vi "virtualDS.vi"(4 "DS Digital Ins":T4, 6 "DS Analog Ins":T3 {"Analog 4" scale=0.0..65535.0; "Analog 3" scale=0.0..65535.0; "Analog 2" scale=0.0..65535.0; "Analog 1" scale=0.0..65535.0}, 7 "Control Byte":T2, 8 "JS 4":T5 {"Axes"."Axis 6" scale=-127.0..127.0; "Axes"."Axis 5" scale=-127.0..127.0; "Axes"."Axis 4" scale=-127.0..127.0; "Axes"."Axis 3" scale=-127.0..127.0; "Axes"."Axis 2" scale=-127.0..127.0; "Axes"."Axis 1" scale=-127.0..127.0}, 9 "JS 3":T5 {"Axes"."Axis 6" scale=-127.0..127.0; "Axes"."Axis 5" scale=-127.0..127.0; "Axes"."Axis 4" scale=-127.0..127.0; "Axes"."Axis 3" scale=-127.0..127.0; "Axes"."Axis 2" scale=-127.0..127.0; "Axes"."Axis 1" scale=-127.0..127.0}, 10 "JS 2":T5 {"Axes"."Axis 6" scale=-127.0..127.0; "Axes"."Axis 5" scale=-127.0..127.0; "Axes"."Axis 4" scale=-127.0..127.0; "Axes"."Axis 3" scale=-127.0..127.0; "Axes"."Axis 2" scale=-127.0..127.0; "Axes"."Axis 1" scale=-127.0..127.0}, 11 "JS 1":T5 {"Axes"."Axis 6" scale=-127.0..127.0; "Axes"."Axis 5" scale=-127.0..127.0; "Axes"."Axis 4" scale=-127.0..127.0; "Axes"."Axis 3" scale=-127.0..127.0; "Axes"."Axis 2" scale=-127.0..127.0; "Axes"."Axis 1" scale=-127.0..127.0}) -> ()   [LabVIEW 2011]
uses:
  joystick.ctl
panel:
  in  "IP Control":T1 {"Team Number" format="%04.0f"}
  out "Packet":string
  out "FRCCommonControlData":string
  out "Packet Number":u16
  in  "stop":bool
  out "length":i32
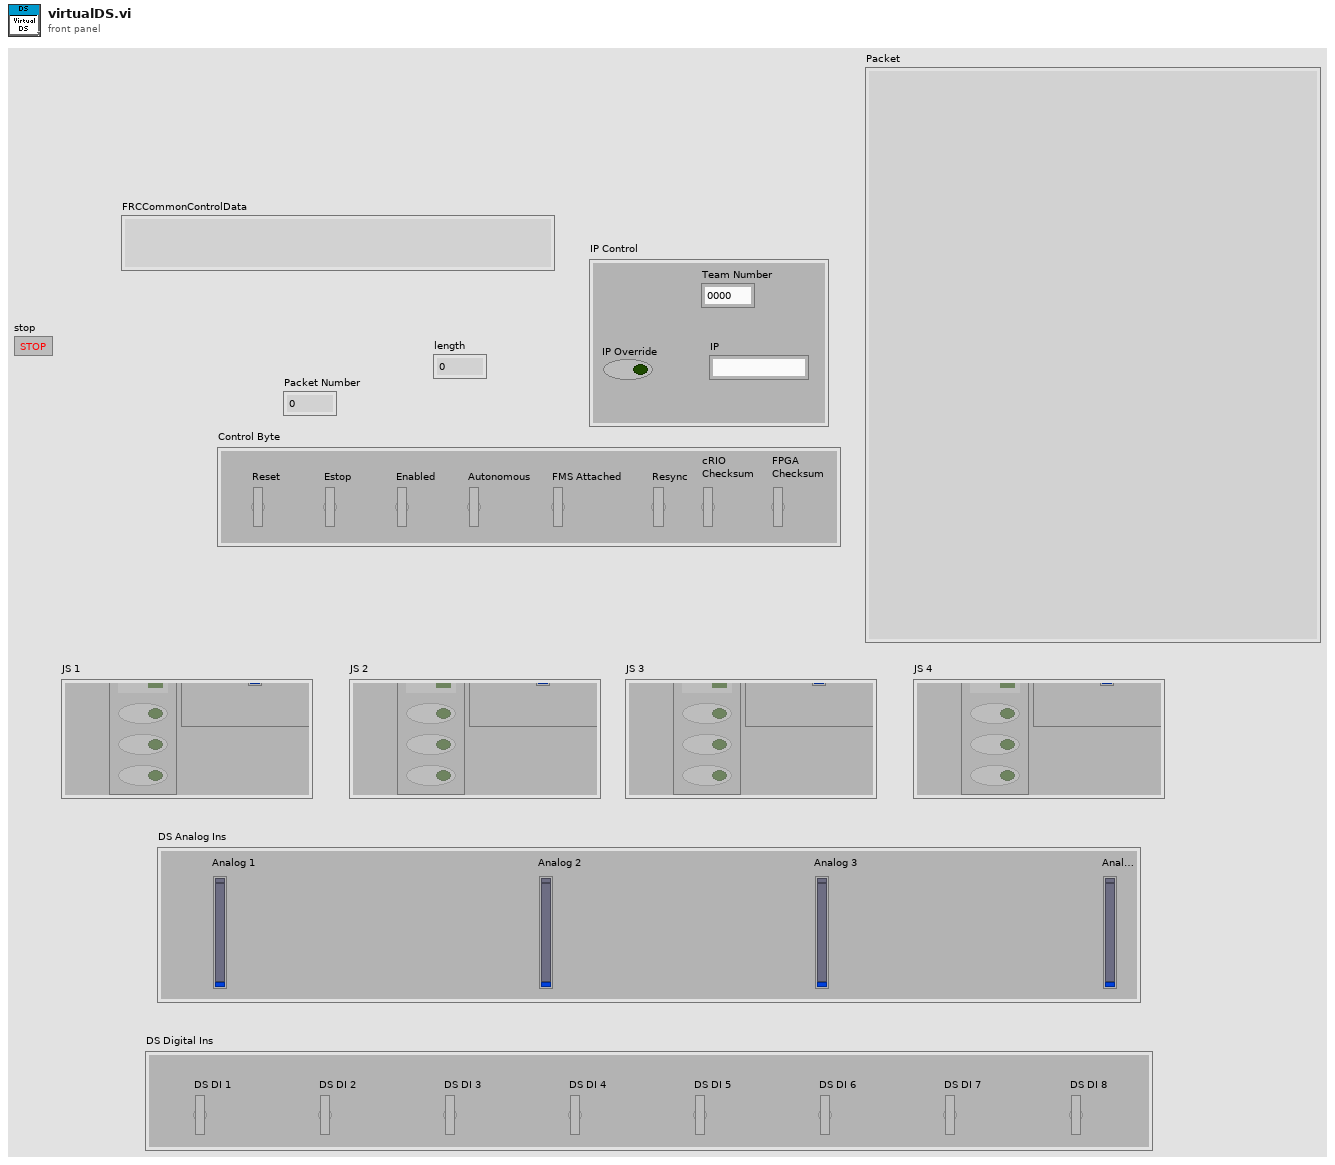
[diagram p1: front panel]
types:
  T1 = cluster{"Team Number":u16, "IP":string, "IP Override":bool}
  T2 = cluster{"Reset":bool, "Estop":bool, "Enabled":bool, "Autonomous":bool, "FMS Attached":bool, "Resync":bool, "cRIO \nChecksum":bool, "FPGA \nChecksum":bool}
  T3 = cluster{"Analog 1":u16, "Analog 2":u16, "Analog 3":u16, "Analog 4":u16}
  T4 = cluster{"DS DI 1":bool, "DS DI 2":bool, "DS DI 3":bool, "DS DI 4":bool, "DS DI 5":bool, "DS DI 6":bool, "DS DI 7":bool, "DS DI 8":bool}
  T5 = typedef "joystick.ctl" = cluster{"Axes":cluster{"Axis 1":u8, "Axis 2":u8, "Axis 3":u8, "Axis 4":u8, "Axis 5":u8, "Axis 6":u8}, "Buttons":bool[]}
  T6 = cluster{"Axis 1":u8, "Axis 2":u8, "Axis 3":u8, "Axis 4":u8, "Axis 5":u8, "Axis 6":u8}
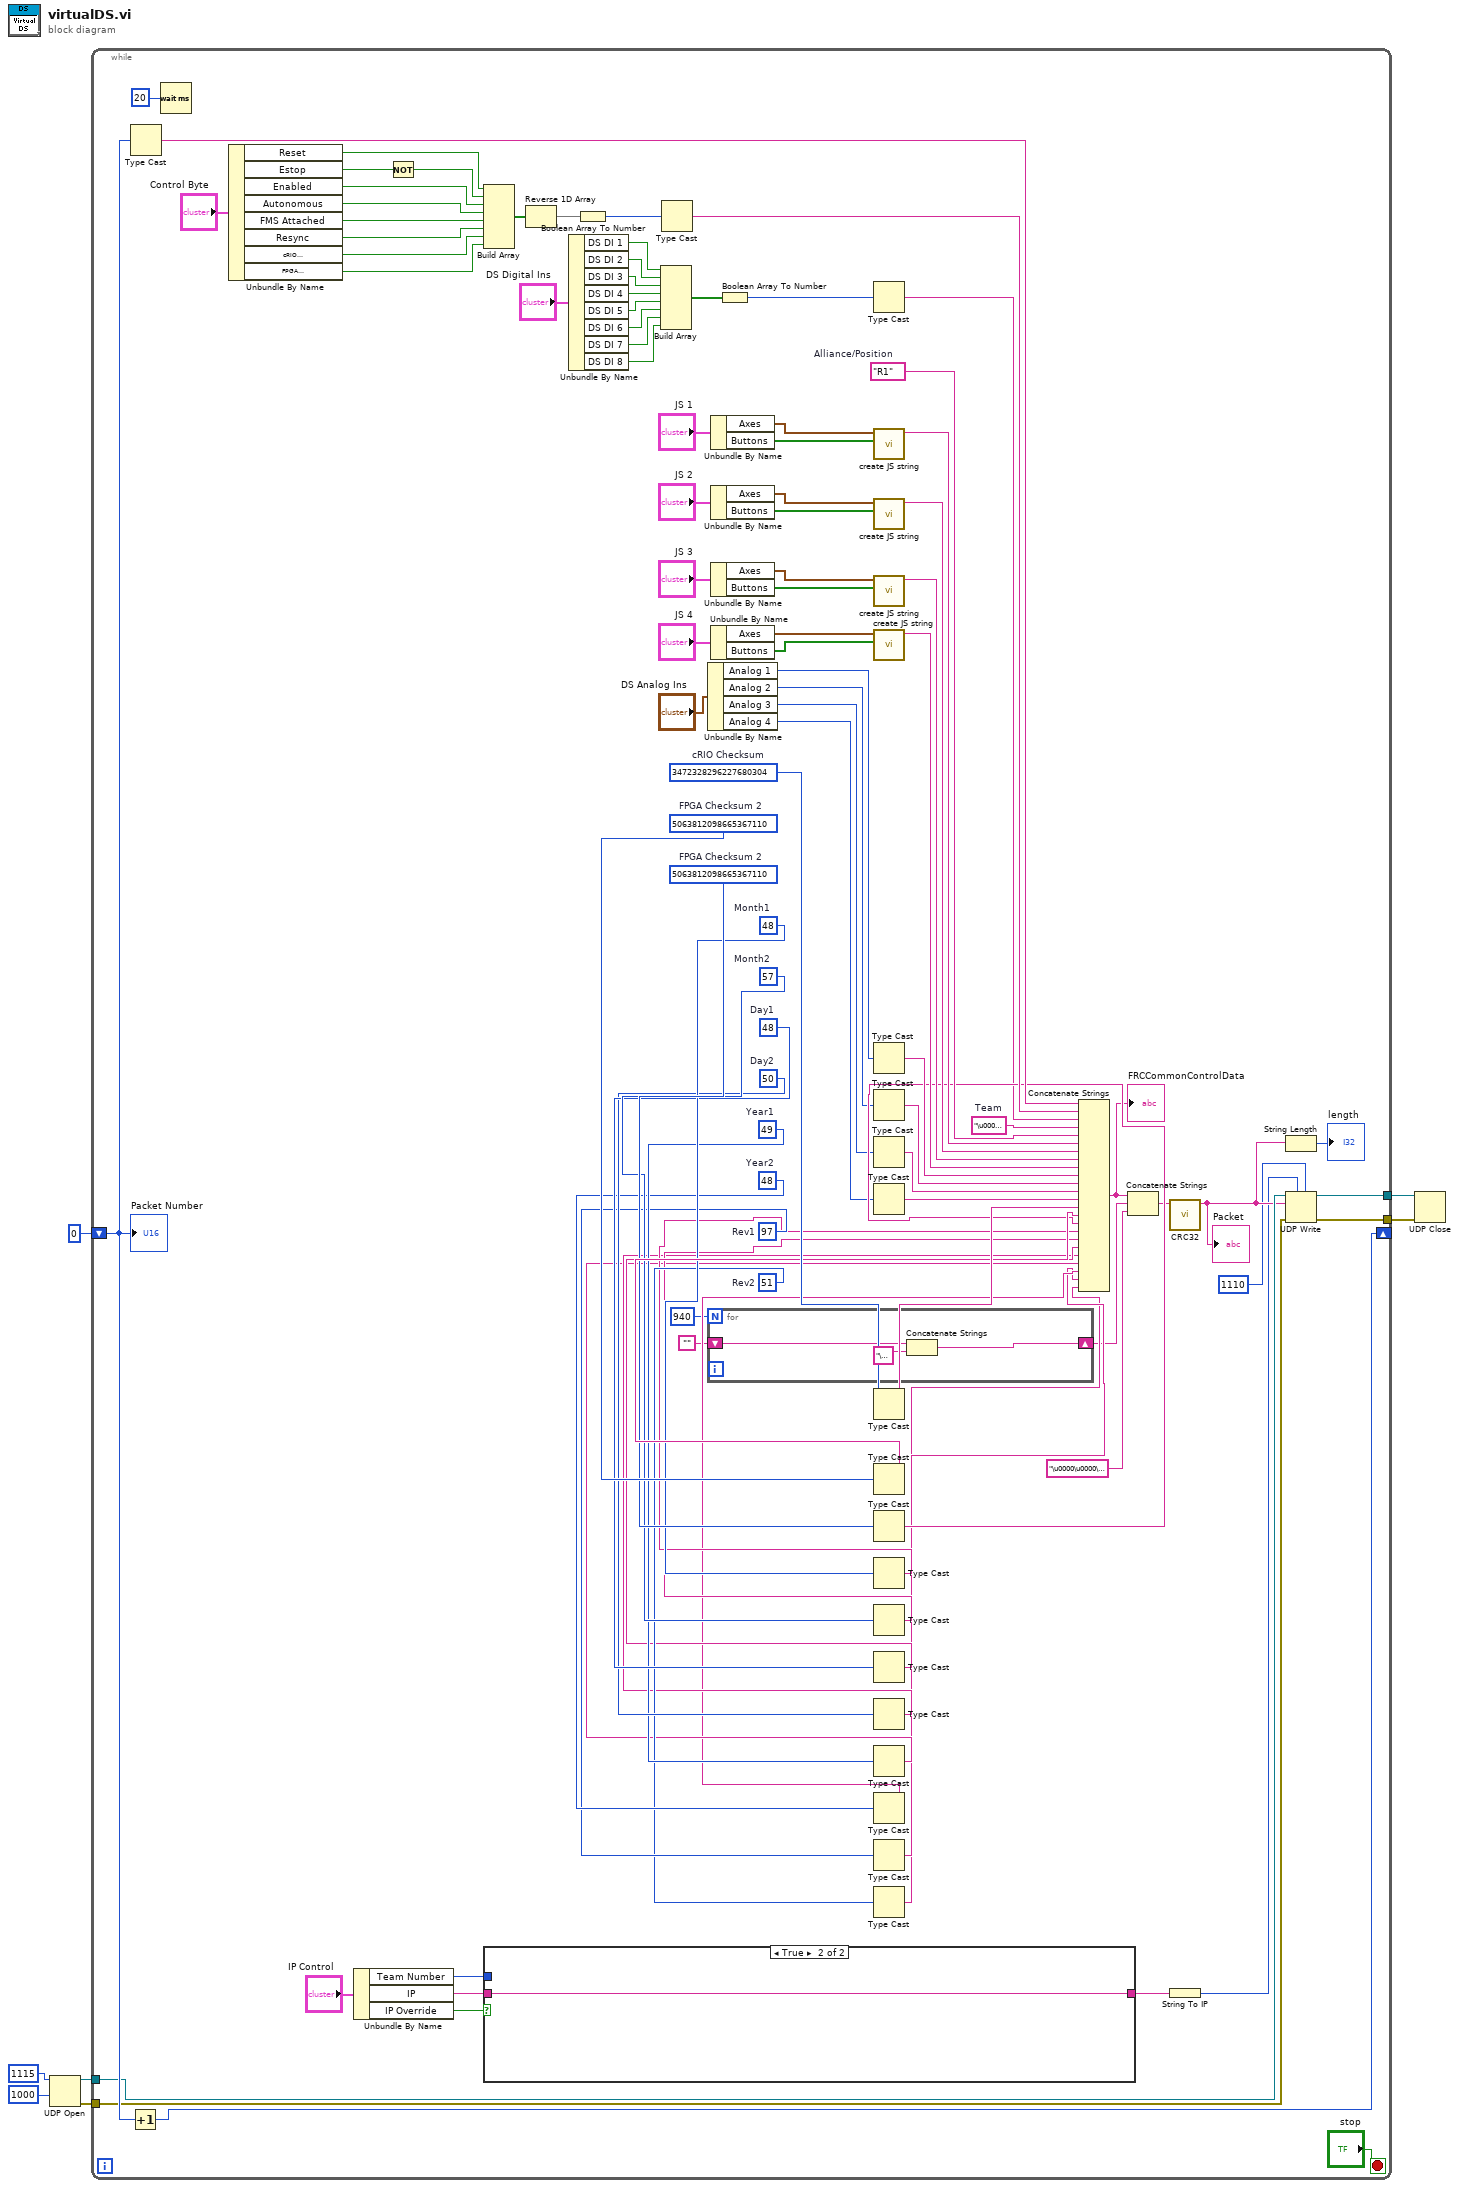
[diagram p0: block diagram]
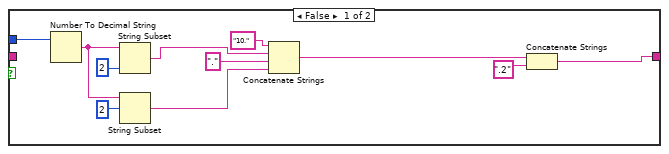
[diagram p2: hidden frame]
diagram:
  n1 = UDP Open(9:1000 ("timeout ms (25000)"), 11:u16 1115 ("port")) -> (port=w4:refnum<k16>, 0:w3:errorcluster)  [unwired: 3 in, 1 out]
  n2 = while {
    shift-right: [w106] -> _
    shift-left: u16 0 -> [w47]
    tunnel: w4 -> [w19]
    tunnel: w3 -> [w18]
    tunnel: [w16] -> w2
    tunnel: [w15] -> w1
    stop <- "stop" stop-if-true
    w66 = u8 51  # Rev2
    w67 = u8 97  # Rev1
    w68 = u8 48  # Year2
    w69 = u8 49  # Year1
    w70 = u8 50  # Day2
    w71 = u8 48  # Day1
    w72 = u8 57  # Month2
    w73 = u8 48  # Month1
    w75 = u64 5063812098665367110  # FPGA Checksum 2
    w77 = u64 5063812098665367110  # FPGA Checksum 2
    w79 = u64 3472328296227680304  # cRIO Checksum
    w100 = "R1"  # Alliance/Position
    w101 = "\u0004\u0012"  # Team
    n3 = Increment(x=w47) -> (x+1=w106:u16)
    n4 = Type Cast(x=w47) -> (*(type *) &x=w104:string)  [unwired: 1 in]
    n5 = Wait (ms)(milliseconds to wait=u32 20) -> ()  [unwired: 1 out]
    n6 = Unbundle By Name("Control Byte") -> ("Reset"=w27:bool, "Estop"=w26:bool, "Enabled"=w25:bool, "Autonomous"=w24:bool, "FMS Attached"=w23:bool, "Resync"=w22:bool, "cRIO \nChecksum"=w21:bool, "FPGA \nChecksum"=w20:bool)
    n7 = Unbundle By Name("IP Control") -> ("Team Number"=w9:u16, "IP"=w8:string, "IP Override"=w10:bool)
    n8 = Not(x=w26) -> (.not. x?=w51:bool)
    n9 = Build Array(w27, w51, w25, w24, w23, w22, w21, w20) -> (w50:bool[])
    n10 = case shown="True" w10 {
      tunnel: [w110 w118] -> w14
      tunnel: w9 -> [w107 _]
      tunnel: w8 -> [_ w118]
      frame False {
        n11 = Number To Decimal String(number=w107) -> (decimal integer string=w108:string)  [unwired: 1 in]
        n12 = String Subset(string=w108, length (rest)=2 ("length (rest)")) -> (substring=w114:string)  [unwired: 1 in]
        n13 = String Subset(string=w108, offset (0)=2) -> (substring=w112:string)  [unwired: 1 in]
        n14 = Concatenate Strings("10." ("string"), w114, "." ("string"), w112) -> (w111:string)
        n15 = Concatenate Strings(w111, ".2" ("string")) -> (w110:string)
      }
      frame True {
      }
    }
    n16 = Reverse 1D Array(array=w50) -> (reversed array=w49:bool[])
    n17 = Unbundle By Name("DS Digital Ins") -> ("DS DI 1"=w44:bool, "DS DI 2"=w43:bool, "DS DI 3"=w42:bool, "DS DI 4"=w41:bool, "DS DI 5"=w40:bool, "DS DI 6"=w39:bool, "DS DI 7"=w37:bool, "DS DI 8"=w38:bool)
    n18 = Boolean Array To Number(Boolean array=w49) -> (number=w105:u8)
    n19 = Build Array(w44, w43, w42, w41, w40, w39, w37, w38) -> (w36:bool[])
    n20 = Type Cast(x=w105) -> (*(type *) &x=w103:string)  [unwired: 1 in]
    n21 = Unbundle By Name("DS Analog Ins") -> ("Analog 1"=w32:u16, "Analog 2"=w31:u16, "Analog 3"=w30:u16, "Analog 4"=w29:u16)
    n22 = for {
      N: 940 -> [_]
      shift-right: [w121] -> w53
      shift-left: "" -> [w120]
      n23 = Concatenate Strings(w120, "\u0000" ("string")) -> (w121:string)
    }
    n24 = Unbundle By Name("JS 1") -> ("Axes"=w94:T6, "Buttons"=w93:bool[])
    n25 = Unbundle By Name("JS 2") -> ("Axes"=w91:T6, "Buttons"=w90:bool[])
    n26 = Unbundle By Name("JS 3") -> ("Axes"=w87:T6, "Buttons"=w86:bool[])
    n27 = Unbundle By Name("JS 4") -> ("Axes"=w85:T6, "Buttons"=w84:bool[])
    n28 = Boolean Array To Number(Boolean array=w36) -> (number=w34:u8)
    n29 = Type Cast(x=w34) -> (*(type *) &x=w35:string)  [unwired: 1 in]
    n30 = call "create JS string.vi"("Buttons"=w93, "Axes"=w94) -> ("Output String"=w99:string)  [unwired: 8 in, 1 out]
    n31 = call "create JS string.vi"("Buttons"=w90, "Axes"=w91) -> ("Output String"=w98:string)  [unwired: 8 in, 1 out]
    n32 = call "create JS string.vi"("Buttons"=w86, "Axes"=w87) -> ("Output String"=w97:string)  [unwired: 8 in, 1 out]
    n33 = call "create JS string.vi"("Buttons"=w84, "Axes"=w85) -> ("Output String"=w96:string)  [unwired: 8 in, 1 out]
    n34 = Type Cast(x=w32) -> (*(type *) &x=w83:string)  [unwired: 1 in]
    n35 = Type Cast(x=w31) -> (*(type *) &x=w82:string)  [unwired: 1 in]
    n36 = Type Cast(x=w30) -> (*(type *) &x=w81:string)  [unwired: 1 in]
    n37 = Type Cast(x=w29) -> (*(type *) &x=w80:string)  [unwired: 1 in]
    n38 = Type Cast(x=w79) -> (*(type *) &x=w78:string)  [unwired: 1 in]
    n39 = Type Cast(x=w77) -> (*(type *) &x=w76:string)  [unwired: 1 in]
    n40 = Type Cast(x=w75) -> (*(type *) &x=w74:string)  [unwired: 1 in]
    n41 = Type Cast(x=w73) -> (*(type *) &x=w65:string)  [unwired: 1 in]
    n42 = Type Cast(x=w72) -> (*(type *) &x=w64:string)  [unwired: 1 in]
    n43 = Type Cast(x=w71) -> (*(type *) &x=w63:string)  [unwired: 1 in]
    n44 = Type Cast(x=w70) -> (*(type *) &x=w62:string)  [unwired: 1 in]
    n45 = Type Cast(x=w69) -> (*(type *) &x=w61:string)  [unwired: 1 in]
    n46 = Type Cast(x=w68) -> (*(type *) &x=w60:string)  [unwired: 1 in]
    n47 = Type Cast(x=w67) -> (*(type *) &x=w59:string)  [unwired: 1 in]
    n48 = Type Cast(x=w66) -> (*(type *) &x=w58:string)  [unwired: 1 in]
    n49 = Concatenate Strings(w104, w103, w35, w101, w100, w99, w98, w97, w96, w83, w82, w81, w80, w78, w76, w74, w65, w64, w63, w62, w61, w60, w59, w58) -> (w56:string)
    "FRCCommonControlData" <- w56
    n50 = Concatenate Strings(w56, w53, "\u0000\u0000\u0000\u0000" ("string")) -> (w48:string)
    n51 = call "CRC32.vi"("In"=w48) -> ("Out"=w17:string)  [unwired: 9 in, 1 out]
    "Packet" <- w17
    n52 = String To IP(1:w14) -> (0:w13:u32)
    n53 = String Length(string=w17) -> (length=→"length":i32)
    n54 = UDP Write(address=w13, port or service name=u16 1110, connection ID=w19, data in=w17, 8:w18) -> (error out=w15:errorcluster, 3:w16:refnum<k16>)  [unwired: 1 in]
    "Packet Number" <- w47
  }
  n55 = UDP Close(connection ID=w2, 8:w1) -> ()  [unwired: 2 out]
